vi "Gamma Moments.vi"(9 "c":dbl=1.0, 10 "b":dbl=1.0) -> (0 "error":i32, 2 "variance":dbl=1.0, 3 "mean":dbl)   [LabVIEW 2014, in "NI_Gmath.lvlib"]
doc: "Returns the expected mean and variance of the random variate X, where X describes the selected distribution type. You must manually select the polymorphic instance to use."
uses:
  NI_Gmath.lvlib
  st_error_code.ctl
panel:
  # "Gamma Moments"
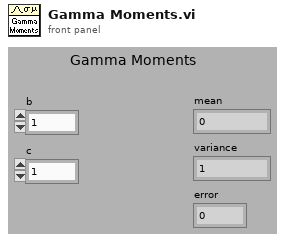
[diagram p1: front panel]
types:
  T1 = typedef "NI_Gmath.lvlib/st_error_code.ctl" = i32
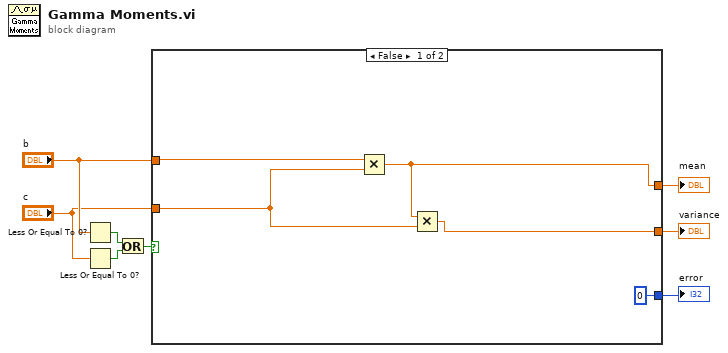
[diagram p0: block diagram]
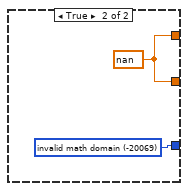
[diagram p2: hidden frame]
diagram:
  n1 = Less Or Equal To 0?(x="b") -> (x <= 0?=w4:bool)
  n2 = Less Or Equal To 0?(x="c") -> (x <= 0?=w5:bool)
  n3 = Or(x=w4, y=w5) -> (x .or. y?=w6:bool)
  n4 = case shown="False" w6 {
    tunnel: "c" -> [w11 _]
    tunnel: [0 ("invalid math domain") w14] -> w8
    tunnel: [w9 w15] -> w7
    tunnel: "b" -> [w12 _]
    tunnel: [w10 w15] -> w1
    frame False {
      n5 = Multiply(x=w12, y=w11) -> (x*y=w9:dbl)
      n6 = Multiply(x=w9, y=w11) -> (x*y=w10:dbl)
    }
    frame True {
      w14 = T1 -20069 items=["invalid math domain"=-20069, "Fourier interpolation size m >= n"=-20070, "empty array"=-20003] ("stat interp error code")
      w15 = nan
    }
  }
  "mean" <- w7
  "error" <- w8
  "variance" <- w1
